vi "GetAllObject.vi"(8 "error in (no error)":errorcluster) -> (0 "error out":errorcluster, 3 "Stand out":refnum<class "Stand.lvclass">)   [LabVIEW 2019, in "Stand.lvclass"]
uses:
  Stand.lvclass
  Database_Postgress_class/Database_Postgress.lvclass
  C:/Users/ANENKOV_V1/Desktop/src/DatabaseInterface_class/DatabaseInterface.lvclass
  Database_Postgress_class/Connection Info.ctl
  Logger_class/Logger.lvclass
  ConfigJSON_class/ConfigJSON.lvclass
  C:/Users/ANENKOV_V1/Desktop/src/ConfigInterface_class/ConfigInterface.lvclass
  Proccess_class/TAGs.ctl
  FPGA_API_class/FPGA API.lvclass
  Modbus_class/ModbusSp.lvclass
  SV_Puplisher_class/SV_Publisher.lvclass
  ConfigJSON_class/ConfigJSON.lvclass/ConfigJSON.ctl
  DatabaseInterface_class/DatabaseInterface.lvclass
  Proccess_class/Proccess.lvclass
panel:
  out "error out 2":errorcluster
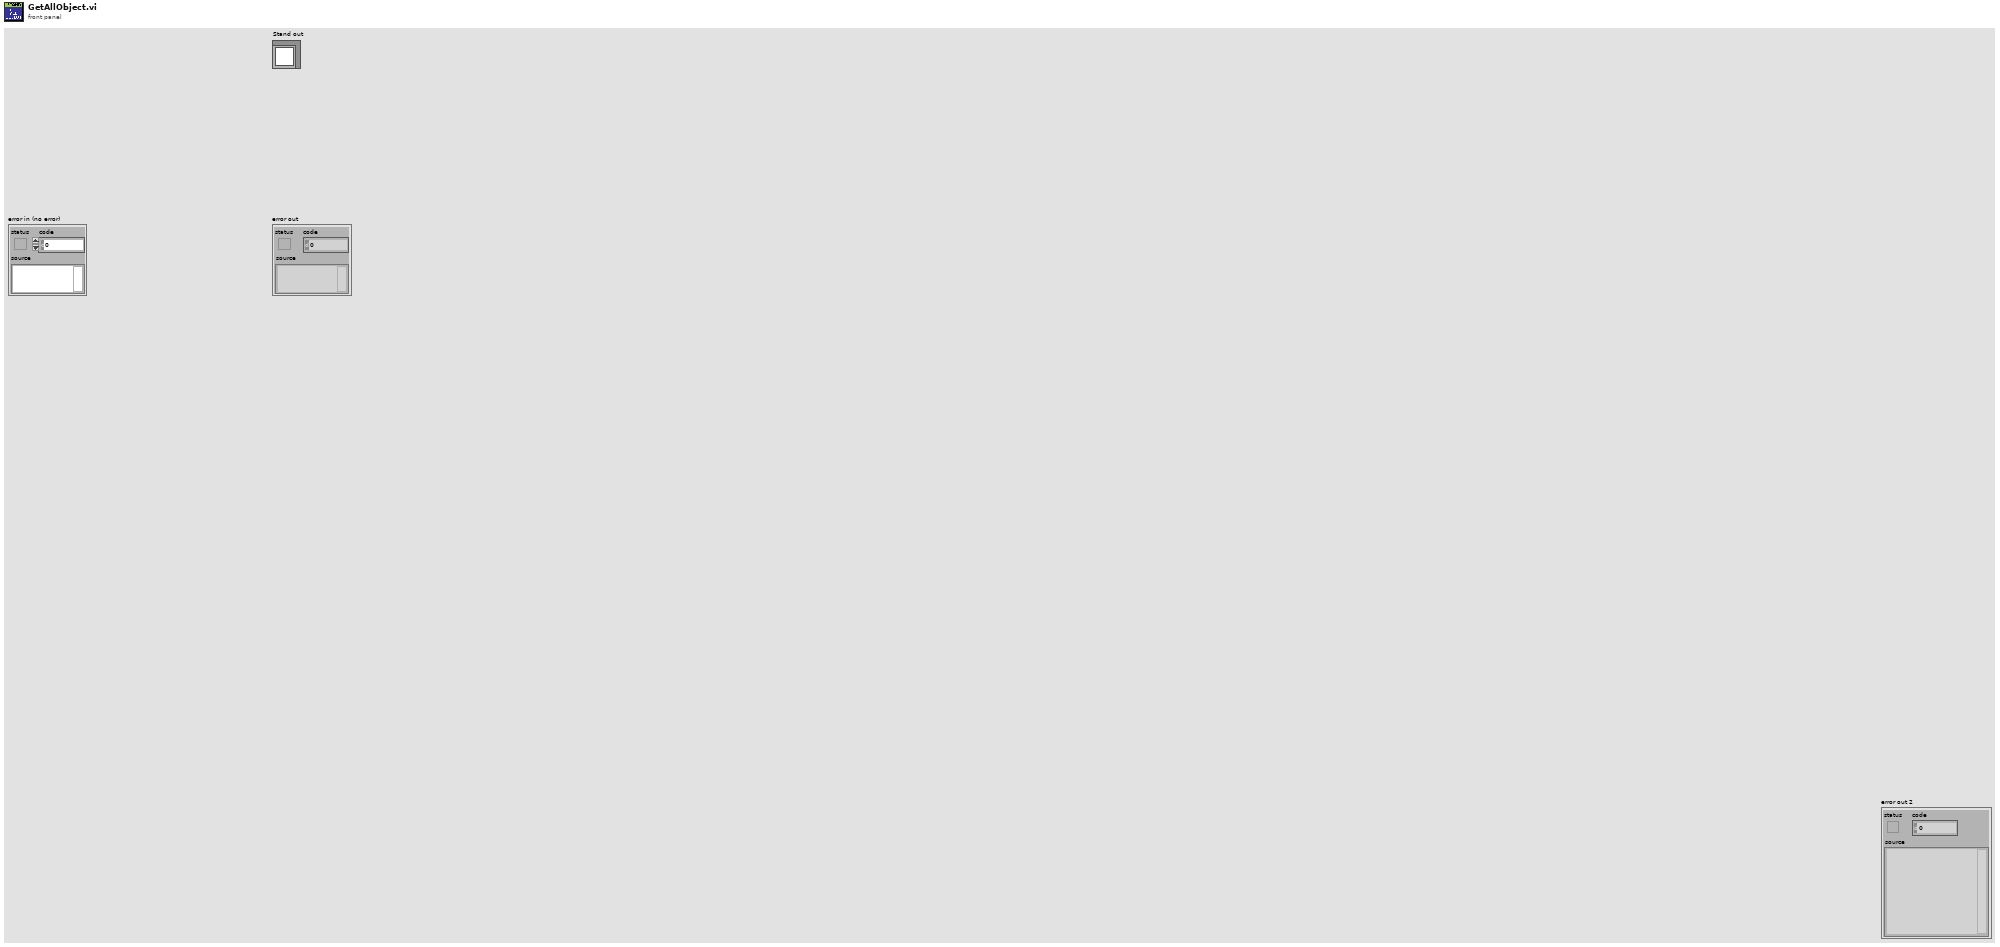
[diagram p1: front panel]
types:
  T1 = typedef "Proccess.lvclass/TAGs.ctl" = cluster{"TAG":string, "PTAG":string, "DESC":string}
  T2 = typedef "DatabaseInterface.lvclass/Connection Info.ctl" = cluster{"IP_Address":string, "Port":u16, "Timeout":i32, "User":string, "Password":string, "Database":string}
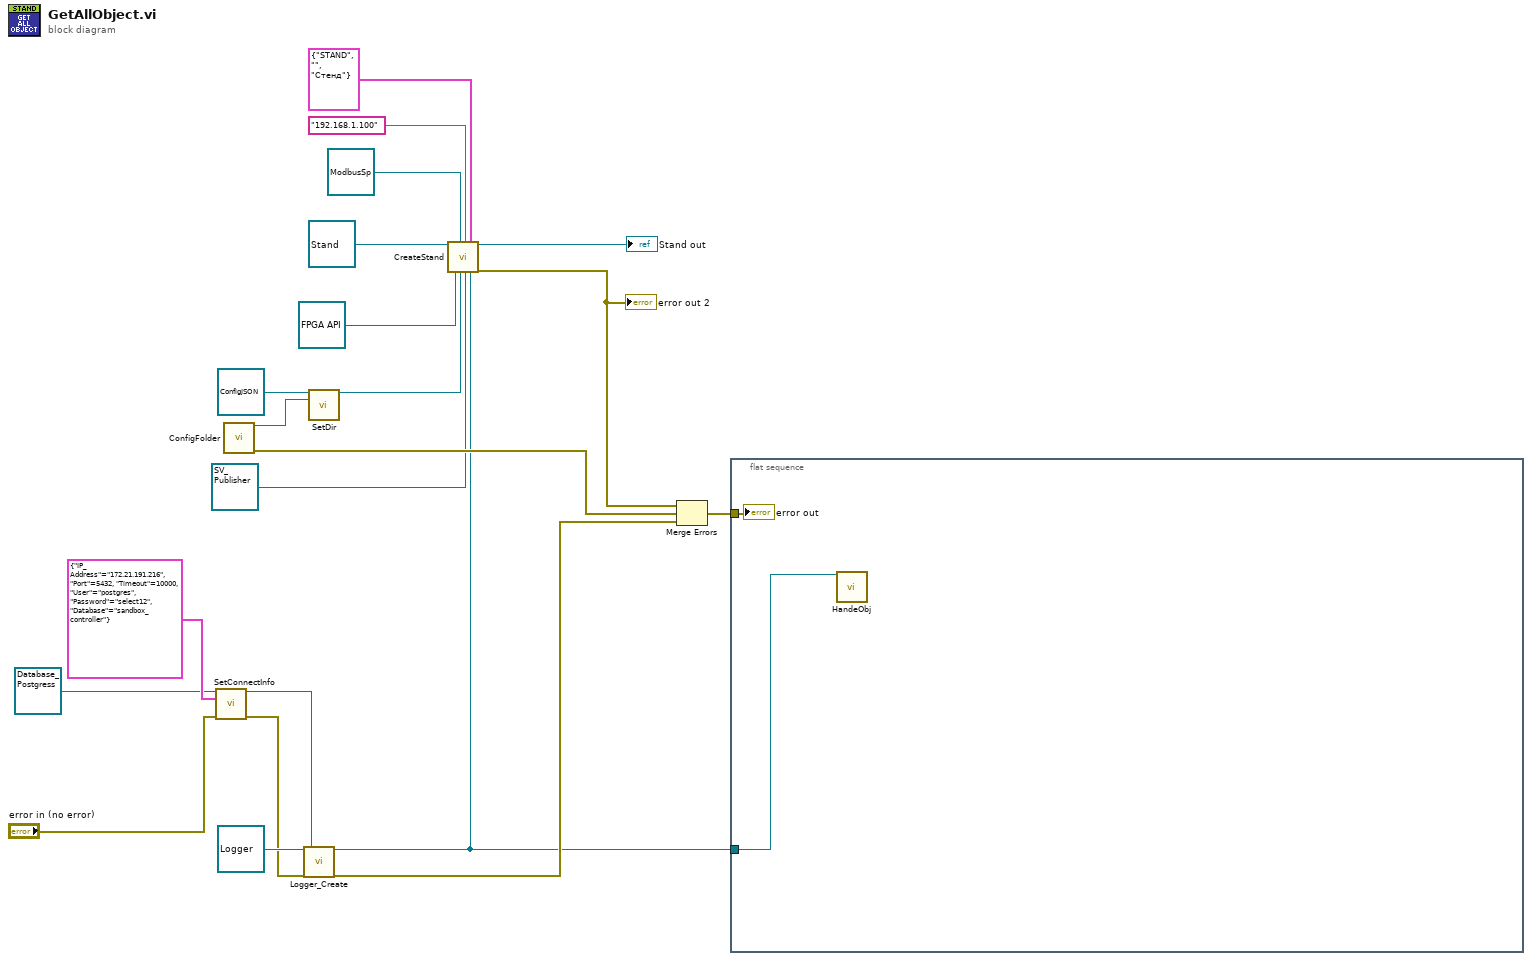
[diagram p0: block diagram]
diagram:
  n1 = call-dynamic "SetConnectInfo.vi"("reference in"=refnum<class "Database_Postgress.lvclass"> refnum, "Connection Info"=T2 {"IP_Address"="172.21.191.216", "Port"=5432, "Timeout"=10000, "User"="postgres", "Password"="select12", "Database"="sandbox_controller"}, "error in (no error)"="error in (no error)") -> ("reference out"=w17:refnum<class "Database_Postgress.lvclass">, "error out"=w16:errorcluster)  [unwired: 11 in]
  n2 = call "ConfigFolder.vi"() -> ("dup path"=w14:path, "error out"=w7:errorcluster)  [unwired: 14 in]
  n3 = call "Logger_Create.vi"("reference in"=refnum<class "Logger.lvclass"> refnum, "error in (no error)"=w16, "DatabaseInterface"=w17) -> ("reference out"=w3:refnum<class "Logger.lvclass">, "error out"=w6:errorcluster)  [unwired: 15 in]
  n4 = call "SetDir.vi"("reference in"=refnum<class "ConfigJSON.lvclass"> refnum ("ConfigJSON"), "Config Dir"=w14) -> ("JSON"=w10:refnum<class "ConfigJSON.lvclass">)  [unwired: 13 in]
  n5 = call "CreateStand.vi"("Stand in"=refnum<class "Stand.lvclass"> refnum, "FPGA API"=refnum<class "FPGA API.lvclass"> refnum, "Modbus"=refnum<class "ModbusSp.lvclass"> refnum, "ConfigInterface"=w10, "NV Addres"="192.168.1.100", "SV_Publisher"=refnum<class "SV_Publisher.lvclass"> refnum, "Tags"=T1 {"TAG"="STAND", "PTAG"="", "DESC"="Стенд"}, "Logger"=w3) -> ("Stand out"=→"Stand out":refnum<class "Stand.lvclass">, "error out"=w8:errorcluster)  [unwired: 10 in]
  "error out 2" <- w8
  n6 = Merge Errors(w8, w7, w6) -> (w5:errorcluster)
  n7 = flat-sequence {
    tunnel: w5 -> [w23]
    tunnel: w3 -> [w22]
    frame #0 {
      n8 = call "HandeObj.vi"("reference in"=w22) -> ()  [unwired: 12 in, 3 out]
      "error out" <- w23
    }
  }
